vi "DCReadXTemplateJK2.vi"(3 ";error in (no error)":errorcluster, 5 ";Type":i32, 6 ";DataIn":string) -> (0 "error out":errorcluster, 1 "Time Stamp":timestamp, 2 ";Data (out)":string)   [LabVIEW 2020]
uses:
  <vilib>/variable/detnetvar/DSV init parameters.ctl
  <vilib>/variable/detnetvar/Network provider/lvedc.dll
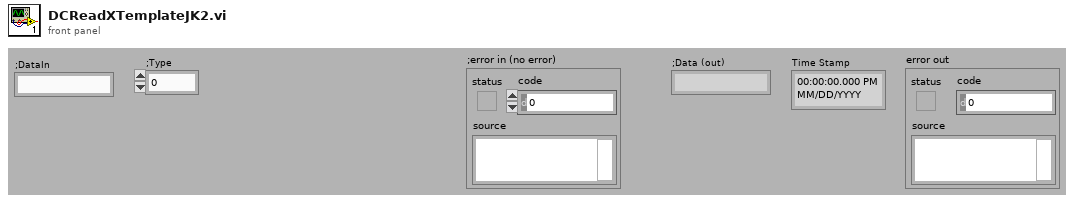
[diagram p1: front panel]
types:
  T1 = typedef "DSV init parameters.ctl" = cluster{"refIndex in":i32, "MAC Address":string, "NodeId":string, "SMB block Offset (us)":i32, "Max Variable Length":i32, "Sub Items":i32, "Item Size (bytes)":u16, "Index":i32, "SMB item Data Offset (bytes)":i32, "Timing Source Name":string, "Node is owner?":bool, "Num Items":i32, "Start Slot (us) ":i32, "GUID":string, "Reserved":string, "Cycle time (us)":i32, "Master?":bool, "Max Overall\n Message Length ":i32, "Version Count":u32, "SMB Start Times (other nodes)":i32[], "Network Speed":enum16{"100 MBit", "1 GBit"}, "SMB Variable":bool}
  T2 = typedef "DCTerminalRefNum.ctl" = cluster{"ID":i32, "GUID":dbl, "Type":enum16{"Terminal"}}
  T3 = typedef "DCTerminalAccessData.ctl" = cluster{"Dif":i32, "Len":i32, "User data":u32}
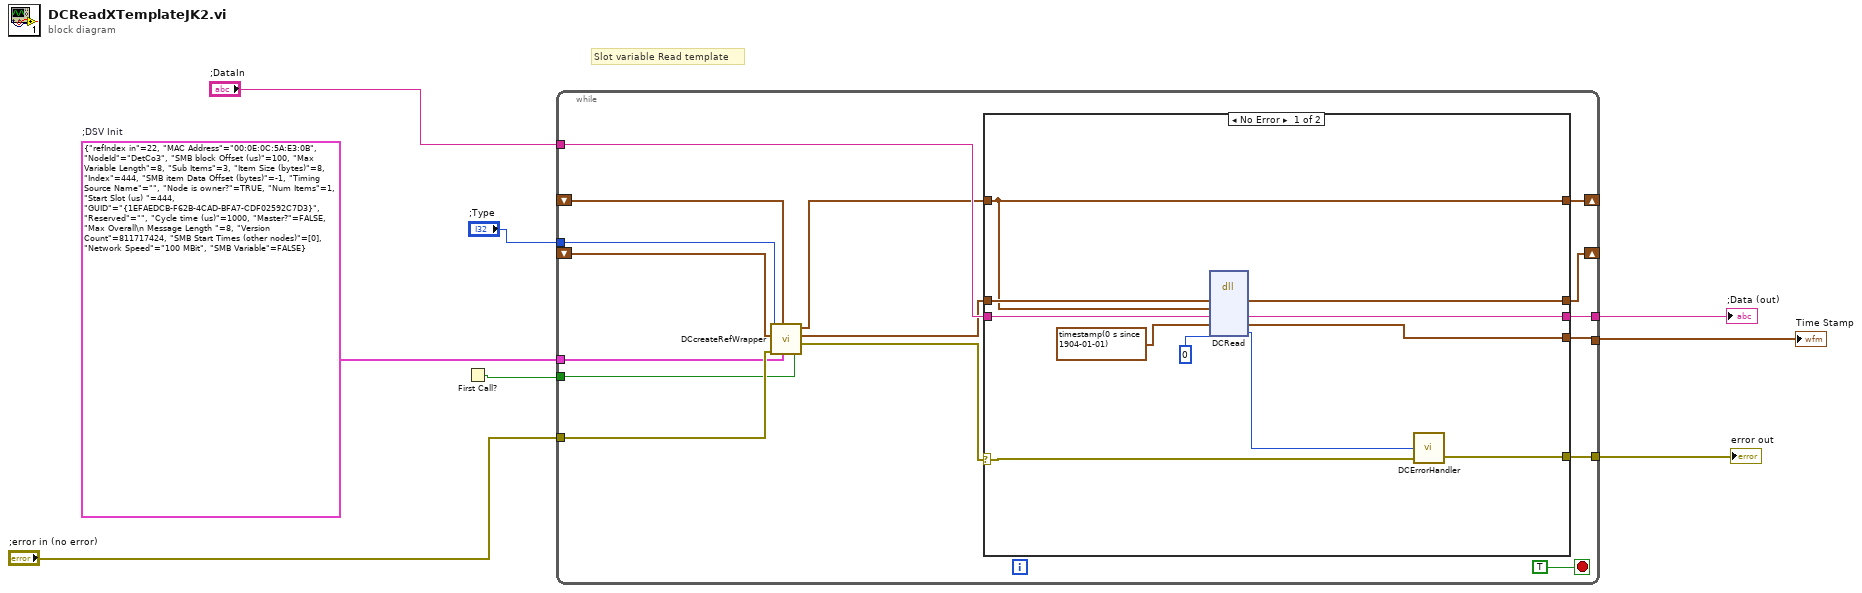
[diagram p0: block diagram]
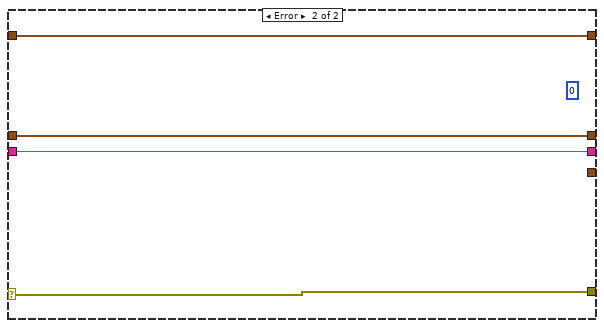
[diagram p2: hidden frame]
diagram:
  w1 = T1 {"refIndex in"=22, "MAC Address"="00:0E:0C:5A:E3:0B", "NodeId"="DetCo3", "SMB block Offset (us)"=100, "Max Variable Length"=8, "Sub Items"=3, "Item Size (bytes)"=8, "Index"=444, "SMB item Data Offset (bytes)"=-1, "Timing Source Name"="", "Node is owner?"=TRUE, "Num Items"=1, "Start Slot (us) "=444, "GUID"="{1EFAEDCB-F62B-4CAD-BFA7-CDF02592C7D3}", "Reserved"="", "Cycle time (us)"=1000, "Master?"=FALSE, "Max Overall\n Message Length "=8, "Version Count"=811717424, "SMB Start Times (other nodes)"=[0], "Network Speed"=enum."100 MBit", "SMB Variable"=FALSE}  # ;DSV Init
  # "Slot variable Read template"
  n1 = First Call?() -> (First Call?: T/F=w6:bool)
  n2 = while {
    tunnel: [w24] -> w7
    tunnel: ";error in (no error)" -> [w17]
    tunnel: ";DataIn" -> [w23]
    tunnel: [w22] -> w4
    shift-right: [w20] -> _
    shift-left: _ -> [w16]
    tunnel: w6 -> [w14]
    tunnel: w1 -> [w15]
    tunnel: [w13] -> w2
    shift-right: [w12] -> _
    shift-left: _ -> [w11]
    tunnel: ";Type" -> [w9]
    stop <- TRUE stop-if-true
    n3 = call <vilib>:"DCcreateRefWrapper.vi"("First Call?: T/F"=w14, ";Init"=w15, ";Terminal Data in"=w11, ";error in (no error)"=w17, "Terminal RefNum (out)"=w16, ";Type"=w9) -> ("Error (out)"=w18:errorcluster, "Terminal RefNum (out) 2"=w19:T2, ";Terminal Data"=w10:T3)  [unwired: 1 in]
    n4 = case shown="No Error" w18 {
      selector: w18 -> [w30 w38]
      tunnel: [w35 w38] -> w24
      tunnel: [w34 w39] -> w20
      tunnel: w10 -> [w27 w36]
      tunnel: w23 -> [w33 w37]
      tunnel: w19 -> [w31 w39]
      tunnel: [w29 w37] -> w22
      tunnel: [w25 _] -> w13
      tunnel: [w27 w36] -> w12
      frame No Error {
        n5 = dll-call lib="e:/penguin/lvdist/win32/export/20.0/20.0.0f0/dist/vi.lib/variable/detnetvar/Network provider/lvedc.dll" fn="DCRead"("Terminal RefNum (out) 2"=w31, ";Terminal Data"=w27, ";DataIn"=w33, "Time Stamp"=timestamp(0 s since 1904-01-01), "status"=0) -> ("Terminal RefNum (out) 2"=w34:T2, ";DataIn"=w29:string, "Time Stamp"=w25:timestamp, "status"=w32:i32)  [unwired: 5 in, 2 out]
        n6 = call <vilib>:"DCErrorHandler.vi"("error in"=w30, "status"=w32) -> ("error out"=w35:errorcluster)  [unwired: 2 in]
      }
      frame Error {
        (unwired) u32 0 ("User data")
      }
    }
  }
  "Time Stamp" <- w2
  "error out" <- w7
  ";Data (out)" <- w4
